vi "Reset Motor Zero.vi"() -> ()   [LabVIEW 2014]
uses:
  ALPHA5 RS485/typedefs/Port Selection Info.ctl
  Delta Robot/Fuji Delta Robot.lvclass/Fuji Delta Robot.ctl
  ALPHA5 RS485/Classes/FujiMotor/FujiMotor.lvclass
  Delta Robot/Fuji Delta Robot.lvclass
  ALPHA5 RS485/ALPHA5 RS485.lvlib
panel:
  in  "index":i32
  out "ENC Pos Before":i32
  out "ENC Pos":i32
  in  "Port Selection Info In":T1={"Port Name"="COM5", "Amplifier Num"=1, "Baud Rate"=38400, "Char Formation"=enum."0"} {"Baud Rate" items=["38400"=38400, "19200"=19200, "9600"=9600, "115200"=0]; "Amplifier Num" max=31}
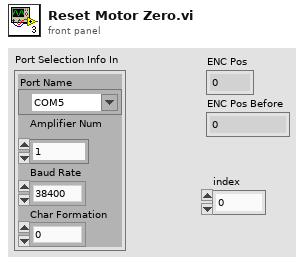
[diagram p1: front panel]
types:
  T1 = typedef "ALPHA5 RS485.lvlib/Port Selection Info.ctl" = cluster{"Port Name":refnum<visa-resource-name>, "Amplifier Num":u8, "Baud Rate":u32, "Char Formation":enum16{"0", "1", "2", "3", "4", "5"}}
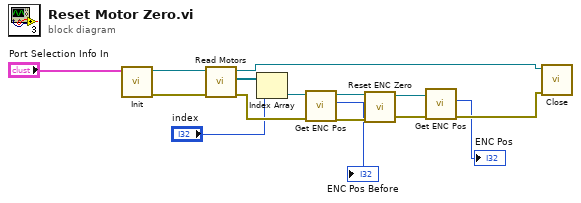
[diagram p0: block diagram]
diagram:
  n1 = call "Init.vi"("Port Selection Info In"="Port Selection Info In") -> ("error out"=w13:errorcluster, "Fuji Delta out"=w14:refnum<class "Fuji Delta Robot.lvclass">)  [unwired: 9 in]
  n2 = call "Read Motors.vi"("error in (no error)"=w13, "Fuji Delta Robot in"=w14) -> ("error out"=w4:errorcluster, "Motors"=w12:refnum<class "FujiMotor.lvclass">[], "Fuji Delta Robot out"=w8:refnum<class "Fuji Delta Robot.lvclass">)  [unwired: 7 in]
  n3 = Index Array(array=w12, index="index") -> (element=w3:refnum<class "FujiMotor.lvclass">)
  n4 = call "Get ENC Pos.vi"("error in (no error)"=w4, "FujiMotor in"=w3) -> ("error out"=w5:errorcluster, "ENC Pos"=→"ENC Pos Before":i32, "FujiMotor out"=w6:refnum<class "FujiMotor.lvclass">)  [unwired: 7 in]
  n5 = call "Reset ENC Zero.vi"("error in (no error)"=w5, "FujiMotor in"=w6) -> ("error out"=w10:errorcluster, "FujiMotor out"=w11:refnum<class "FujiMotor.lvclass">)  [unwired: 8 in]
  n6 = call "Get ENC Pos.vi"("error in (no error)"=w10, "FujiMotor in"=w11) -> ("error out"=w9:errorcluster, "ENC Pos"=→"ENC Pos":i32)  [unwired: 7 in, 1 out]
  n7 = call "Close.vi"("error in (no error)"=w9, "Fuji Delta in"=w8) -> ()  [unwired: 9 in, 1 out]
